vi "TriggerShell.vi"() -> ()   [LabVIEW 2014]
uses:
  <vilib>/measure/mamon.llb/Trigger Detection for 1 Channel.vi
  <vilib>/measure/NI_MAPro.lvlib
panel:
  out "trigger location (normal program)":dbl format="%#_2g"
  out "Trigger Locations":i32[](array[numeric])
  out "trigger detected?":bool
  in  "Trigger":bool
  in  "Stop Graphing":bool
  in  "stop":bool
  out "Waveform Graph":dynamicdata(graph)
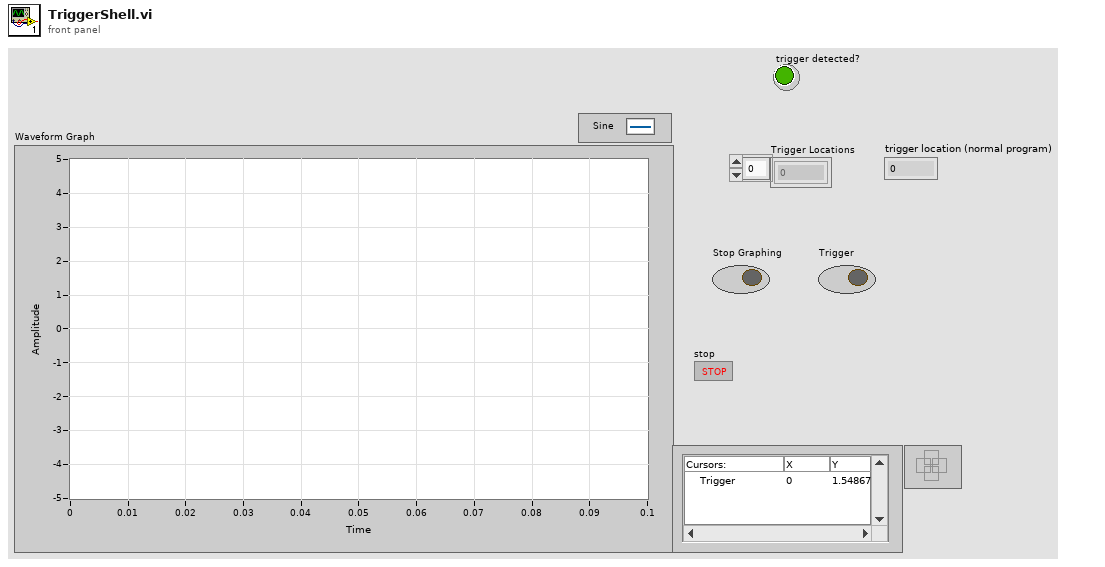
[diagram p1: front panel]
types:
  T1 = cluster{"Cursor.Cursor Y":dbl, waveform(dbl), dbl, "location mode":u16, "error in (no error)":errorcluster, "trigger slope":u16}
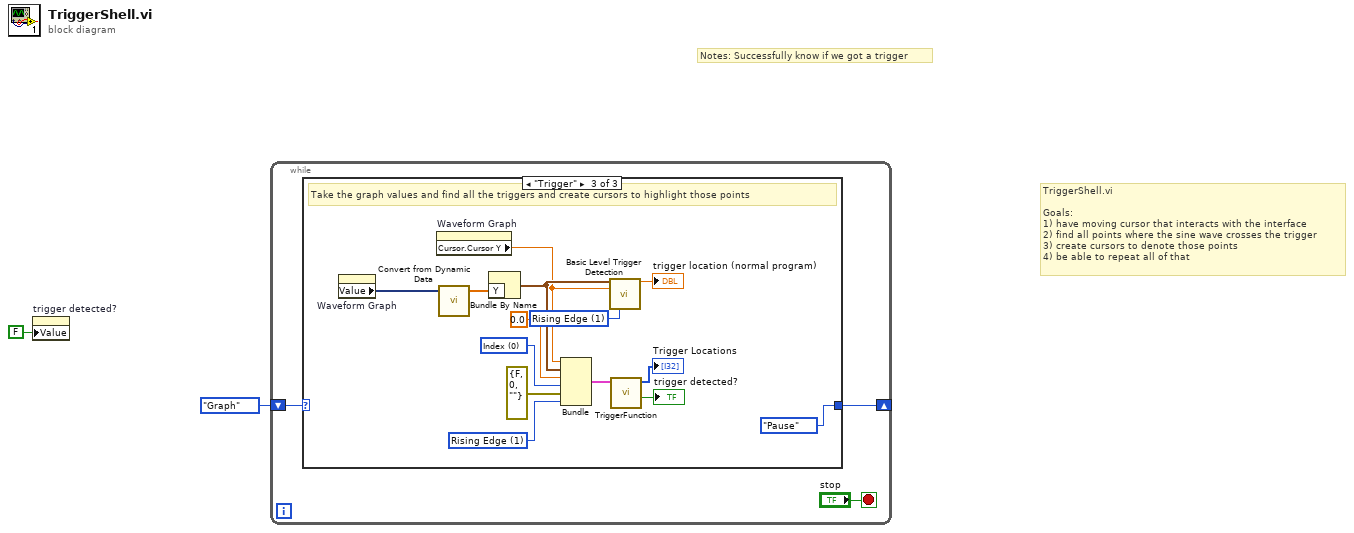
[diagram p0: block diagram]
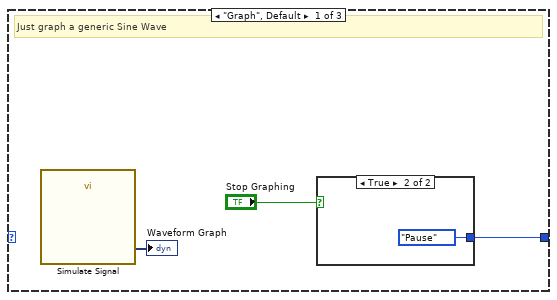
[diagram p2: hidden frame]
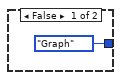
[diagram p3: hidden frame]
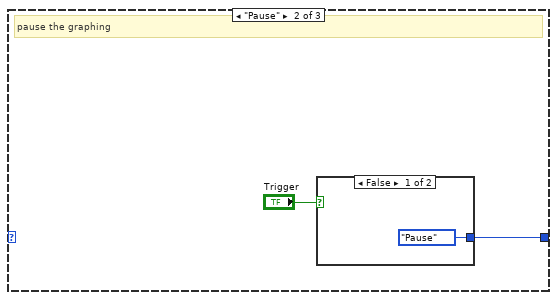
[diagram p4: hidden frame]
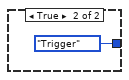
[diagram p5: hidden frame]
diagram:
  # "Notes: Successfully know if we got a trigger"
  # "TriggerShell.vi\n\nGoals:\n1) have moving cursor that interacts with the interface\n2) find all points where the sine wave crosses the trigger\n3) create cursors to denote those points\n4) be able to repeat all of that"
  n1 = property on="trigger detected?" class="Bool (strict)"("Value"=FALSE ("trigger detected?")) -> ()  [unwired: 2 in, 2 out]
  n2 = while {
    shift-right: [w3] -> _
    shift-left: enum16{"Graph", "Trigger", "Pause"}."Graph" -> [w4]
    stop <- "stop" stop-if-true
    n3 = case shown="\"Trigger\"" w4 {
      tunnel: [w6 w11 enum16{"Graph", "Trigger", "Pause"}."Pause"] -> w3
      frame "Graph", Default {
        # "Just graph a generic Sine Wave"
        n4 = call "Simulate Signal"() -> ("Sine"=→"Waveform Graph":dynamicdata)  [unwired: 14 in, 1 out]
        n5 = case shown="True" "Stop Graphing" {
          tunnel: [enum16{"Graph", "Trigger", "Pause"}."Graph" enum16{"Graph", "Trigger", "Pause"}."Pause"] -> w6
          frame False {
          }
          frame True {
          }
        }
      }
      frame "Pause" {
        # "pause the graphing"
        n6 = case shown="False" "Trigger" {
          tunnel: [enum16{"Graph", "Trigger", "Pause"}."Pause" enum16{"Graph", "Trigger", "Pause"}."Trigger"] -> w11
          frame False {
          }
          frame True {
          }
        }
      }
      frame "Trigger" {
        w16 = u16 1 items=["Falling Edge", "Rising Edge"] ("trigger slope")
        w22 = u16 1 items=["Falling Edge", "Rising Edge"] ("trigger slope")
        w24 = u16 0 items=["Index", "Time"] ("location mode")
        # "Take the graph values and find all the triggers and create cursors to highlight those points"
        n7 = property on="Waveform Graph" class="WFGraph (strict)"() -> ("Value"=w27:dynamicdata)  [unwired: 2 in, 2 out]
        n8 = property on="Waveform Graph" class="WFGraph (strict)"() -> ("Cursor.Cursor Y"=w17:dbl)  [unwired: 2 in, 2 out]
        n9 = call "Convert from Dynamic Data"("Dynamic Data Type"=w27) -> ("Array"=w26:dbl[])  [unwired: 3 in]
        n10 = Bundle By Name("Y"=w26) -> (w18:waveform(dbl))  [unwired: 1 in]
        n11 = Bundle("Cursor.Cursor Y"=w17, w18, 0.0, "location mode"=w24, "error in (no error)"=errorcluster {"status"=FALSE, "code"=0, "source"=""}, "trigger slope"=w22) -> (w21:T1)  [unwired: 1 in]
        n12 = call-poly <vilib>:"Basic Level Trigger Detection.vi"("signal in"=w18, "level"=w17, "trigger slope"=w16) -> ("trigger location"=→"trigger location (normal program)":dbl)  [unwired: 10 in, 2 out]
        n13 = call "TriggerFunction.vi"("Input Cluster"=w21) -> ("trigger detected?"=→"trigger detected?":bool, "Trigger Locations"=→"Trigger Locations":i32[])  [unwired: 7 in, 1 out]
      }
    }
  }
